vi "fgv_DSP_return.vi"(7 "cmd":T2, 8 "error in (no error)":errorcluster, 11 "return":T1) -> (0 "error out":errorcluster, 3 "return 2":T1)   [LabVIEW 2019]
uses:
  _ctrl/rw.ctl
  _ctrl/DSP_retrun.ctl
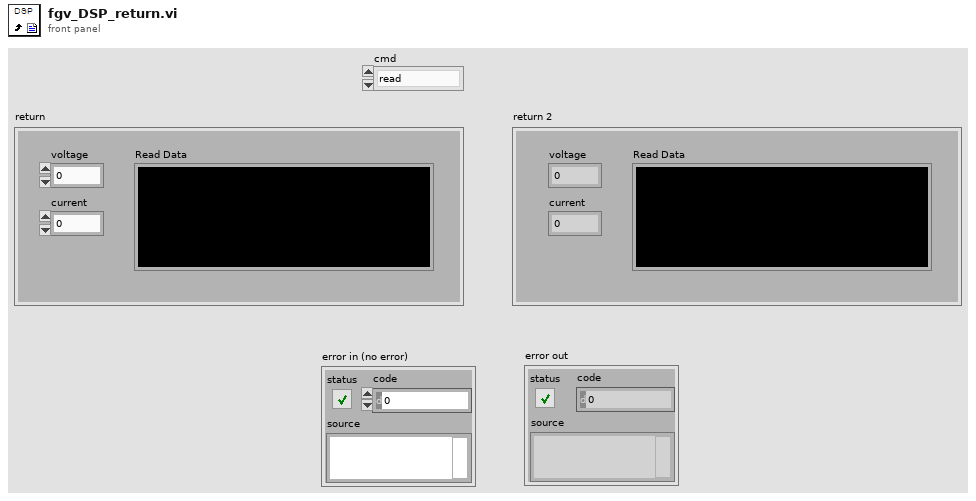
[diagram p1: front panel]
types:
  T1 = typedef "DSP_retrun.ctl" = cluster{"voltage":dbl, "current":dbl, "Read Data":string}
  T2 = typedef "rw.ctl" = enum16{"read", "write"}
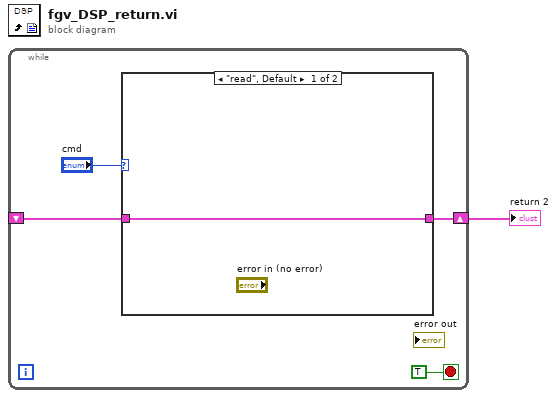
[diagram p0: block diagram]
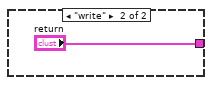
[diagram p2: hidden frame]
diagram:
  n1 = while {
    shift-right: [w3] -> w1
    shift-left: _ -> [w2]
    stop <- TRUE stop-if-true
    n2 = case shown="\"read\", Default" "cmd" {
      tunnel: [w6 "return"] -> w3
      tunnel: w2 -> [w6 _]
      frame "read", Default {
      }
      frame "write" {
      }
    }
  }
  "return 2" <- w1
